vi "PositiveNegativeSpliter.vi"(2 "Offset":dbl[](array[numeric]), 3 "Inputs":dbl[](array[numeric])) -> (0 "Negative":dbl[](array[numeric]), 1 "Positive":dbl[](array[numeric]))   [LabVIEW 2016]
panel:
  out "Positive":T1(graph)
  out "Negative":T1(graph)
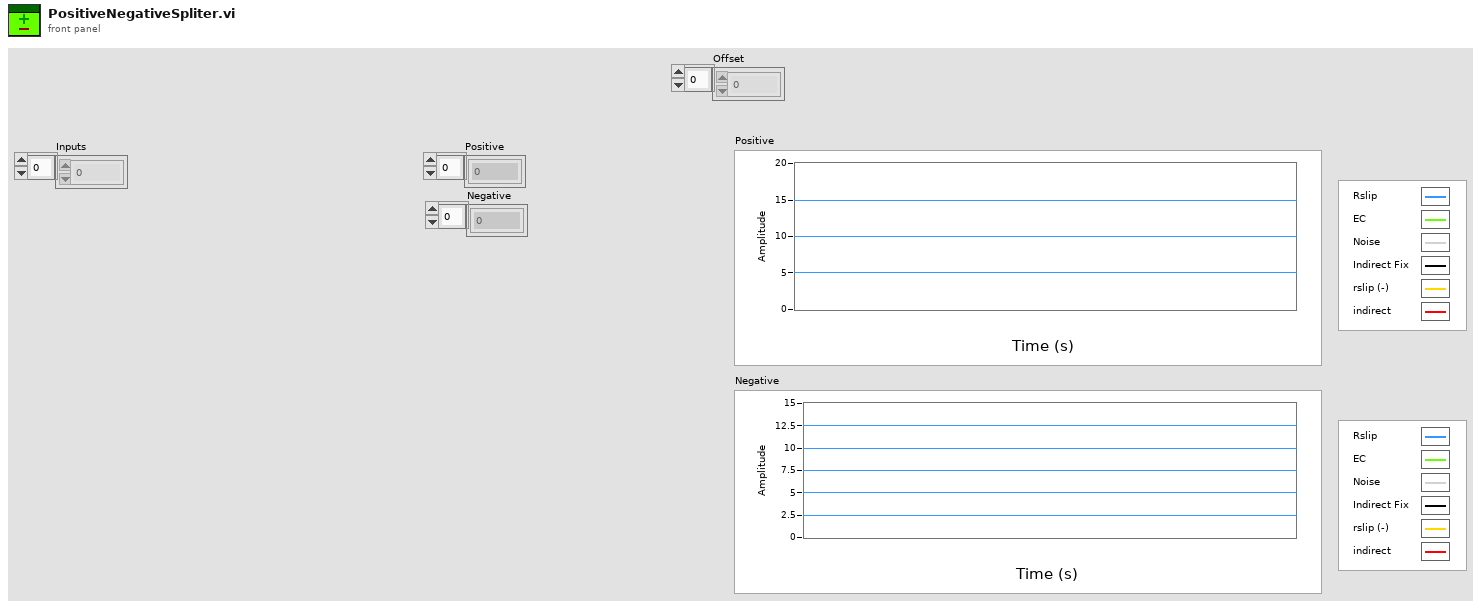
[diagram p1: front panel]
types:
  T1 = cluster{"[0]":dbl, "[1]":dbl, "[2]":dbl, "[3]":dbl, "[4]":dbl, "[5]":dbl, "[6]":dbl, "[7]":dbl, "[8]":dbl}
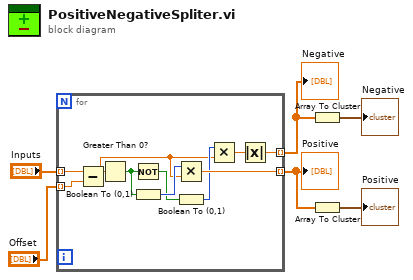
[diagram p0: block diagram]
diagram:
  n1 = for {
    tunnel: "Inputs" -> [w13] mode=indexing
    tunnel: [w15] -> w2 mode=indexing
    tunnel: [w11] -> w4 mode=indexing
    tunnel: "Offset" -> [w7] mode=indexing
    n2 = Subtract(x=w13, y=w7) -> (x-y=w8:dbl)
    n3 = Greater Than 0?(x=w8) -> (x > 0?=w10:bool)
    n4 = Not(x=w10) -> (.not. x?=w9:bool)
    n5 = Boolean To (0,1)(Boolean=w10) -> (0, 1=w16:i16)
    n6 = Multiply(x=w16, y=w8) -> (x*y=w15:dbl)
    n7 = Boolean To (0,1)(Boolean=w9) -> (0, 1=w14:i16)
    n8 = Multiply(x=w14, y=w8) -> (x*y=w12:dbl)
    n9 = Absolute Value(x=w12) -> (abs(x)=w11:dbl)
  }
  "Positive" <- w2
  "Negative" <- w4
  n10 = Array To Cluster(array=w4) -> (cluster=→"Negative":T1)
  n11 = Array To Cluster(array=w2) -> (cluster=→"Positive":T1)
